vi "VITemplate-Reg Events.vi"(11 "error in (no error)":errorcluster) -> (15 "error out":errorcluster)   [LabVIEW 2015]
panel:
  in  "temp":cluster{}
  in  "dummy in":void[](array[numeric])
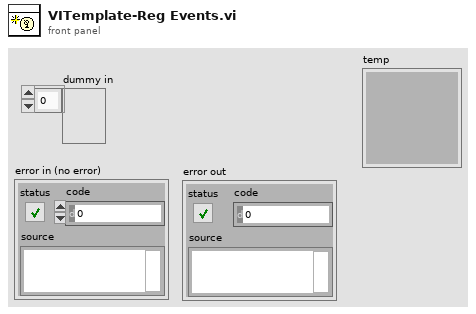
[diagram p1: front panel]
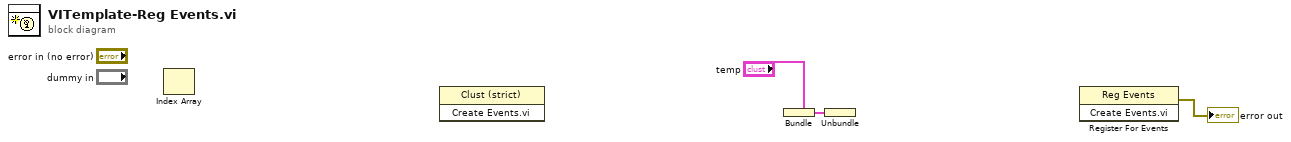
[diagram p0: block diagram]
diagram:
  n1 = Index Array() -> ()  [unwired: 2 in, 1 out]
  n2 = invoke class="Clust (strict)" method="Create Events.vi"() -> ()  [unwired: 3 in, 3 out]
  n3 = Bundle(cluster="temp") -> (w3:cluster{void})  [unwired: 1 in]
  n4 = Unbundle(w3) -> ()  [unwired: 1 out]
  n5 = register-events() -> (error out=→"error out":errorcluster)  [unwired: 3 in, 1 out]
